vi "Acquire.vi"(8 "error in (no error)":errorcluster, 9 "Data Queue":refnum<queue>, 10 "Data Notifier":refnum<notifier>, 11 "Hardware Resources in":T1) -> (0 "error out":errorcluster, 3 "Hardware Resources out":T1)   [LabVIEW 2013, in "Logging Acquisition.lvlib"]
doc: "Perform the acquisition. Replace the contents of this diagram with calls to acquisition hardware."
uses:
  Logging Acquisition.lvlib
  Hardware Configuration.ctl
  Signal Type.ctl
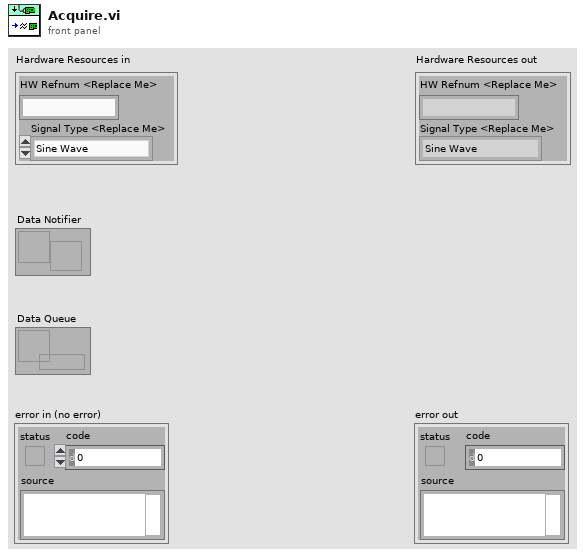
[diagram p1: front panel]
types:
  T1 = typedef "Logging Acquisition.lvlib/Hardware Configuration.ctl" = cluster{"HW Refnum <Replace Me>":string, "Signal Type <Replace Me>":T2}
  T2 = typedef "Logging Acquisition.lvlib/Signal Type.ctl" = enum16{"Sine Wave", "Square with Noise"}
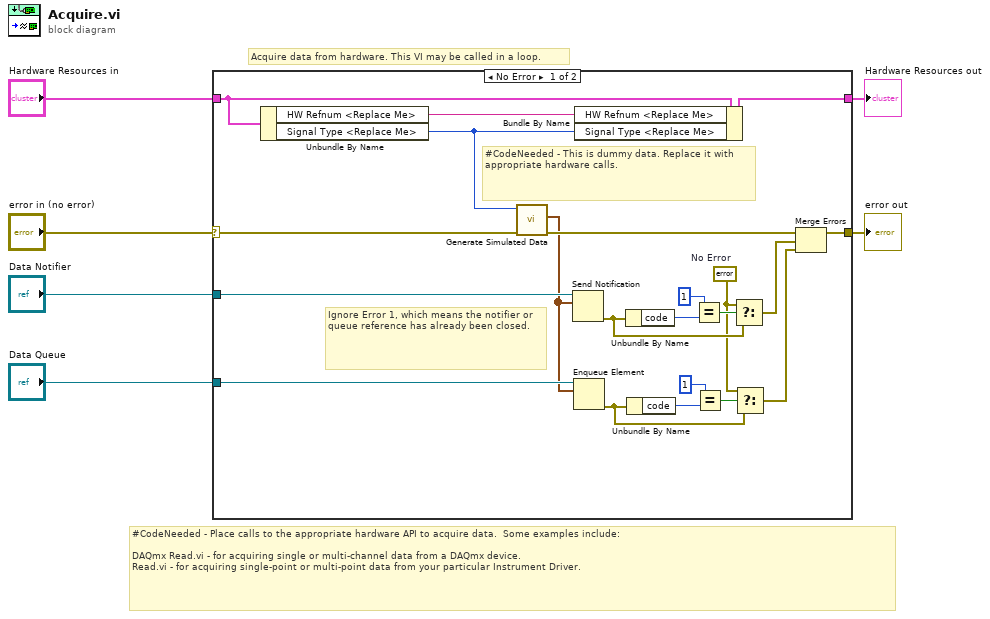
[diagram p0: block diagram]
diagram:
  # "Acquire data from hardware. This VI may be called in a loop."
  # "#CodeNeeded - Place calls to the appropriate hardware API to acquire data.  Some examples include:\n\nDAQmx Read.vi - for acquiring single or multi-channel data from a DAQmx device.\nRead.vi - for acquiring single-point or multi-point data from your particular Instrument Driver."
  n1 = case shown="No Error" "error in (no error)" {
    selector: "error in (no error)" -> [w25 w28]
    tunnel: [w26 w28] -> w5
    tunnel: "Hardware Resources in" -> [w21 w29]
    tunnel: [w27 w29] -> w3
    tunnel: "Data Notifier" -> [w20 _]
    tunnel: "Data Queue" -> [w9 _]
    frame No Error {
      w7 = errorcluster {"status"=FALSE, "code"=0, "source"=""}  # No Error
      # "Ignore Error 1, which means the notifier or queue reference has already been closed."
      # "#CodeNeeded - This is dummy data. Replace it with appropriate hardware calls."
      n2 = Unbundle By Name(w21) -> ("HW Refnum <Replace Me>"=w22:string, "Signal Type <Replace Me>"=w23:T2)
      n3 = call "Generate Simulated Data.vi"("error in (no error)"=w25, "Signal Type"=w23) -> ("error out"=w24:errorcluster, "Graph Data"=w8:waveform(dbl)[])  [unwired: 8 in]
      n4 = Send Notification(notification=w8, notifier=w20) -> (error out=w16:errorcluster)  [unwired: 1 in, 1 out]
      n5 = Enqueue Element(queue=w9, element=w8) -> (error out=w14:errorcluster)  [unwired: 2 in, 2 out]
      n6 = Bundle By Name(cluster=w21, "HW Refnum <Replace Me>"=w22, "Signal Type <Replace Me>"=w23) -> (w27:T1)
      n7 = Unbundle By Name(w16) -> ("code"=w19:i32)
      n8 = Unbundle By Name(w14) -> ("code"=w11:i32)
      n9 = Equal?(x=1, y=w19) -> (x = y?=w17:bool)
      n10 = Equal?(x=1, y=w11) -> (x = y?=w13:bool)
      n11 = Select(t=w7, s=w17, f=w16) -> (s? t:f=w15:errorcluster)
      n12 = Select(t=w7, s=w13, f=w14) -> (s? t:f=w10:errorcluster)
      n13 = Merge Errors(w24, w15, w10) -> (w26:errorcluster)
    }
    frame Error {
    }
  }
  "Hardware Resources out" <- w3
  "error out" <- w5
